vi "mainControlAuto.vi"(8 "error IO":errorcluster, 11 "QueueCluste":T1) -> (3 "error IO 2":errorcluster)   [LabVIEW 2017, in "LibraryGcode.lvlib"]
uses:
  LibraryGcode.lvlib
  control/Queue/QueueCMDandPOS.ctl
  control/Queue/TypeDataPOS.ctl
  control/stateCmdUpdatePara.ctl
  <vilib>/Platform/TimedLoop/XDataNode/timing_clust.ctl
  <vilib>/Platform/TimedLoop/XDataNode/nitl_modes.ctl
  <vilib>/Platform/TimedLoop/XDataNode/wakeup.ctl
  control/stateAutoMode.ctl
  ControlGlobal/stateModeDevice.ctl
  variableGlobal/StartAutoandGcode.vi
  <vilib>/Platform/TimedLoop/XDataNode/XDataNode.xnode
  <vilib>/Platform/TimedLoop/XDataNode/XDNodeRunTimeDep.lvlib
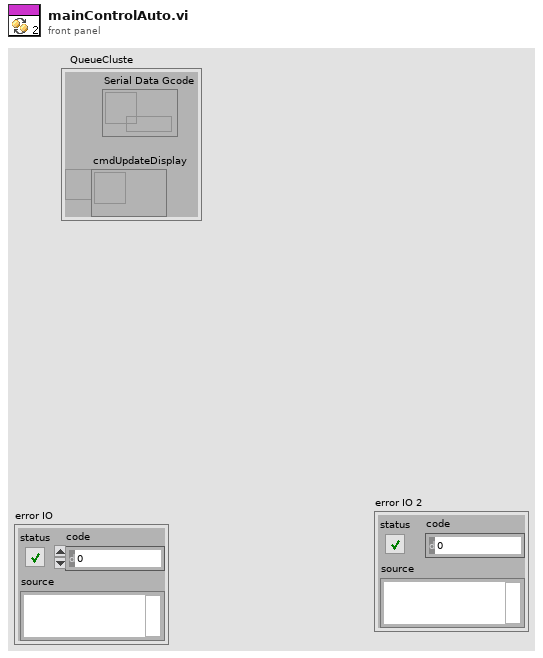
[diagram p1: front panel]
types:
  T1 = typedef "LibraryGcode.lvlib/QueueCMDandPOS.ctl" = cluster{"Serial Data Gcode":refnum<queue>, "cmdUpdateDisplay":refnum<queue>}
  T2 = typedef "LibraryGcode.lvlib/stateAutoMode.ctl" = enum16{"init", "wait", "running", "end"}
  T3 = typedef "XDNodeRunTimeDep.lvlib/timing_clust.ctl" = cluster{"Expected End [f-1]":u64, "Actual End [f-1]":u64, "Finished Late? [f-1]":bool, "Expected End [i-1]":u64, "Actual End [i-1]":u64, "Finished Late? [i-1]":bool, "Expected Start [i]":u64, "Actual Start [i]":u64, "Expected Start [f]":u64, "Actual Start [f]":u64, "Source Name":string, "Structure Name":string, "Period":i64, "Deadline":i64, "Offset":i64, "Start":i64, "Priority":i32, "Timeout":i32, "Mode":T4, "Wakeup Reason":T5, "Error":errorcluster, "Source Type":string, "Secondary Source Type":string, "Global End Time":u64, "Global Start Time":u64, "Frame Duration":u64, "Iteration Duration":u64, "Assigned CPU":i32, "I/O Scan Engine Mode":u32}
  T4 = typedef "XDNodeRunTimeDep.lvlib/nitl_modes.ctl" = enum32{"No Change", "Process missed periods, maintain original phase", "Discard missed periods, maintain original phase", "Process missed periods, ignore original phase", "Discard missed periods, ignore original phase"}
  T5 = typedef "XDNodeRunTimeDep.lvlib/wakeup.ctl" = enum32{"Normal", "Aborted", "Asynchronous wakeup", "Timing source error", "Timed loop error", "Timeout"}
  T6 = typedef "stateModeDevice.ctl" = enum16{"Auto", "Menu", "WaitAutoFinish", "Config", "initAuto"}
  T7 = typedef "LibraryGcode.lvlib/stateBoardFirmware.ctl" = enum16{"Running", "Waiting", "Pos", "IDLE"}
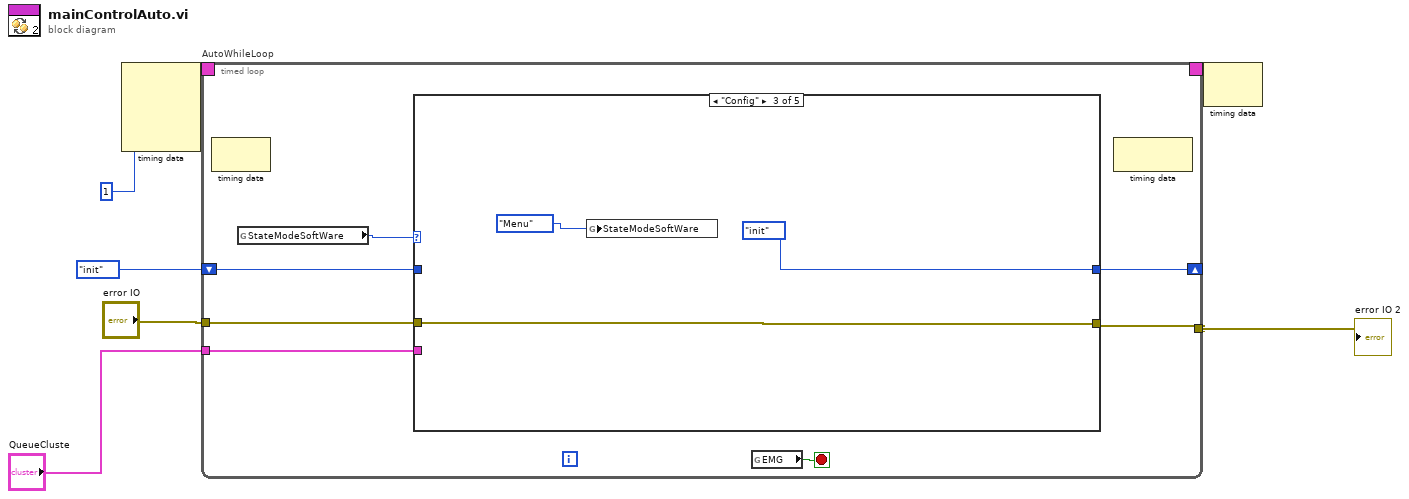
[diagram p0: block diagram]
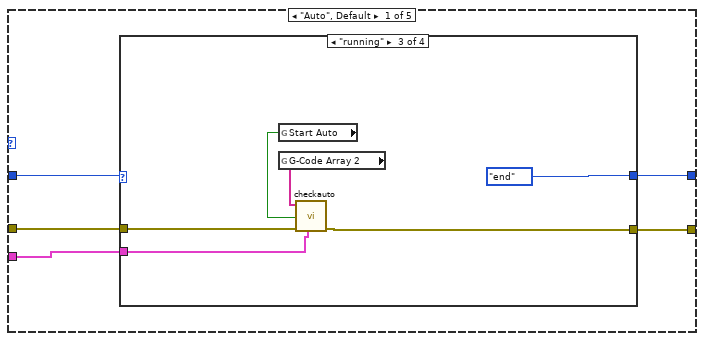
[diagram p2: hidden frame]
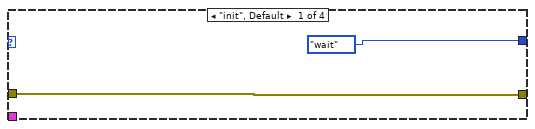
[diagram p3: hidden frame]
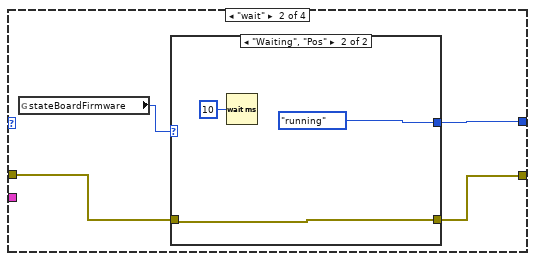
[diagram p4: hidden frame]
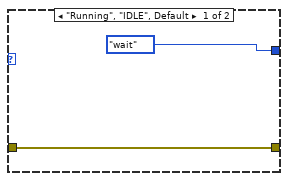
[diagram p5: hidden frame]
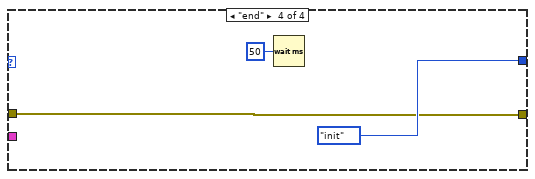
[diagram p6: hidden frame]
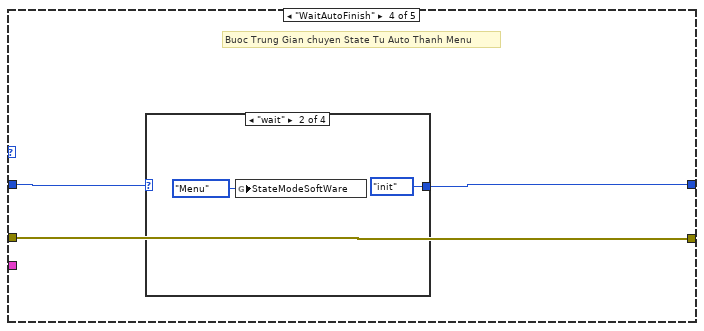
[diagram p8: hidden frame]
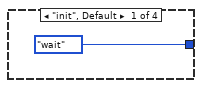
[diagram p9: hidden frame]
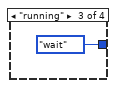
[diagram p10: hidden frame]
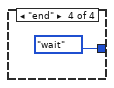
[diagram p11: hidden frame]
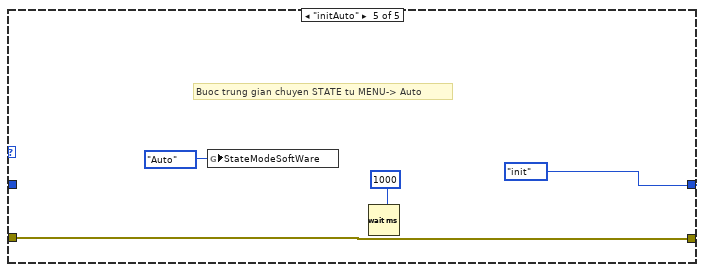
[diagram p12: hidden frame]
diagram:
  n1 = node-c288(1 ("Processor")) -> (w7:T3)  [unwired: 3 in]
  n2 = timed-loop "AutoWhileLoop" {
    shift-right: [w13] -> _
    shift-left: stateAutoMode."init" -> [w14]
    tunnel: "error IO" -> [w12]
    tunnel: "QueueCluste" -> [w8]
    tunnel: [w11] -> w2
    timing: w7 -> [_]
    timing-out: [_] -> w6
    stop <- w9 stop-if-true
    n3 = node-c288() -> ()  [unwired: 1 in, 1 out]
    n4 = global read "StartAutoandGcode.vi" "StateModeSoftWare"() -> (w10:T6)
    n5 = case shown="\"Config\"" w10 {
      tunnel: w14 -> [w17 w43 _ w47 _]
      tunnel: [w21 w43 stateAutoMode."init" w49 stateAutoMode."init"] -> w13
      tunnel: w8 -> [w19 _ _ _ _]
      tunnel: w12 -> [w18 w42 w45 w48 w58]
      tunnel: [w20 w42 w45 w48 w58] -> w11
      frame "Auto", Default {
        n6 = case shown="\"running\"" w17 {
          tunnel: [stateAutoMode."wait" ("stateAuto out") w26 stateAutoMode."end" ("stateAuto out") stateAutoMode."init" ("stateAuto out")] -> w21
          tunnel: [w22 w25 w38 w39] -> w20
          tunnel: w19 -> [_ _ w37 _]
          tunnel: w18 -> [w22 w24 w35 w39]
          frame "init", Default {
          }
          frame "wait" {
            n7 = global read "StartAutoandGcode.vi" "stateBoardFirmware"() -> (w27:T7)
            n8 = case shown="\"Waiting\", \"Pos\"" w27 {
              tunnel: [stateAutoMode."wait" stateAutoMode."running"] -> w26
              tunnel: [w28 w30] -> w25
              tunnel: w24 -> [w28 w30]
              frame "Running", "IDLE", Default {
              }
              frame "Waiting", "Pos" {
                n9 = Wait (ms)(milliseconds to wait=u32 10) -> ()  [unwired: 1 out]
              }
            }
          }
          frame "running" {
            n10 = global read "StartAutoandGcode.vi" "Start Auto"() -> (w36:bool)
            n11 = global read "StartAutoandGcode.vi" "G-Code Array 2"() -> (w34:string[])
            n12 = call "checkauto.vi"("G-Code Array"=w34, "Start Auto"=w36, "error in (no error)"=w35, "queue"=w37) -> ("error out"=w38:errorcluster)  [unwired: 6 in]
          }
          frame "end" {
            n13 = Wait (ms)(milliseconds to wait=u32 50) -> ()  [unwired: 1 out]
          }
        }
      }
      frame "Menu" {
      }
      frame "Config" {
        n14 = global write "StartAutoandGcode.vi" "StateModeSoftWare"(stateModeDevice."Menu" ("statusMode")) -> ()
      }
      frame "WaitAutoFinish" {
        # "Buoc Trung Gian chuyen State Tu Auto Thanh Menu"
        n15 = case shown="\"wait\"" w47 {
          tunnel: [stateAutoMode."wait" stateAutoMode."init" stateAutoMode."wait" stateAutoMode."wait"] -> w49
          frame "init", Default {
          }
          frame "wait" {
            n16 = global write "StartAutoandGcode.vi" "StateModeSoftWare"(stateModeDevice."Menu" ("statusMode")) -> ()
          }
          frame "running" {
          }
          frame "end" {
          }
        }
      }
      frame "initAuto" {
        # "Buoc trung gian chuyen STATE tu MENU-> Auto"
        n17 = global write "StartAutoandGcode.vi" "StateModeSoftWare"(stateModeDevice."Auto" ("statusMode")) -> ()
        n18 = Wait (ms)(milliseconds to wait=u32 1000) -> ()  [unwired: 1 out]
      }
    }
    n19 = global read "StartAutoandGcode.vi" "EMG"() -> (w9:bool)
    n20 = node-c288() -> ()  [unwired: 1 in, 1 out]
  }
  "error IO 2" <- w2
  n21 = node-c288(w6) -> ()  [unwired: 1 out]
